vi "IsFull.vi"(11 "POTTypedCircularBuffer in":refnum<class "POTTypedCircularBuffer.lvclass">) -> (2 "Full?":bool, 3 "POTTypedCircularBuffer out":refnum<class "POTTypedCircularBuffer.lvclass">)   [LabVIEW 2024, in "POTTypedCircularBuffer.lvclass"]
uses:
  POTTypedCircularBuffer.lvclass
  POTTypedCircularBuffer.lvclass/POTTypedCircularBuffer.ctl
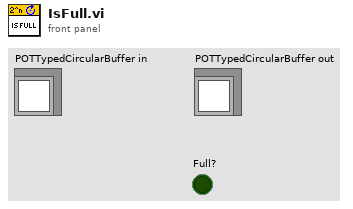
[diagram p1: front panel]
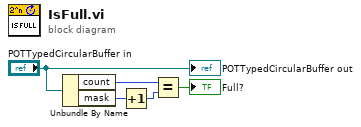
[diagram p0: block diagram]
diagram:
  n1 = Unbundle By Name("POTTypedCircularBuffer in") -> ("count"=w2:i32, "mask"=w3:i32)
  n2 = Increment(x=w3) -> (x+1=w1:i32)
  n3 = Equal?(x=w2, y=w1) -> (x = y?=→"Full?":bool)
  "POTTypedCircularBuffer out" <- "POTTypedCircularBuffer in"
